vi "GetParam.vi"(8 "error in (no error)":errorcluster caption="entrée d'erreur (pas d'erreur)", 11 "GroupShuffleSplit.lvclass":refnum<class "GroupShuffleSplit.lvclass">) -> (0 "error out":errorcluster caption="sortie d'erreur", 2 "GroupShuffleSplit":T1={"n_splits"=5, "test_size"="0,2", "train_size"="None", "random_state"=-1} {"random_state" min=-1}, 3 "GroupShuffleSplit.lvclass":refnum<class "GroupShuffleSplit.lvclass">)   [LabVIEW 2020, in "GroupShuffleSplit.lvclass"]
doc: "Get Parameters"
uses:
  GroupShuffleSplit.lvclass
  GroupShuffleSplit.lvclass/GroupShuffleSplit.ctl
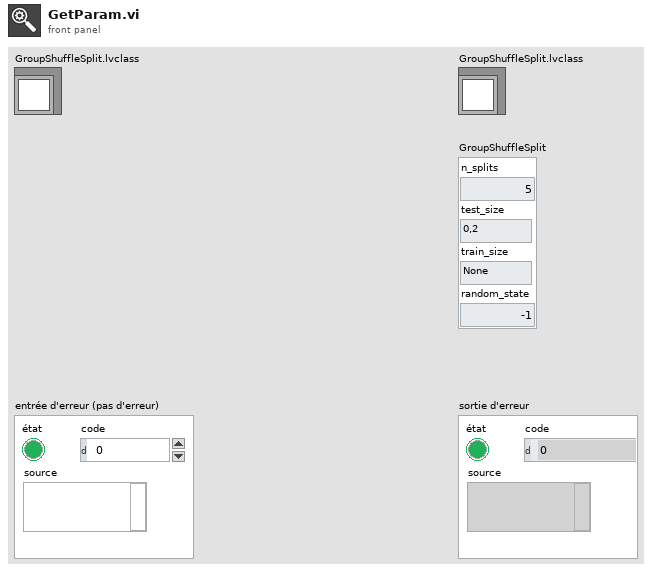
[diagram p1: front panel]
types:
  T1 = cluster{"n_splits":i32, "test_size":string, "train_size":string, "random_state":i32}
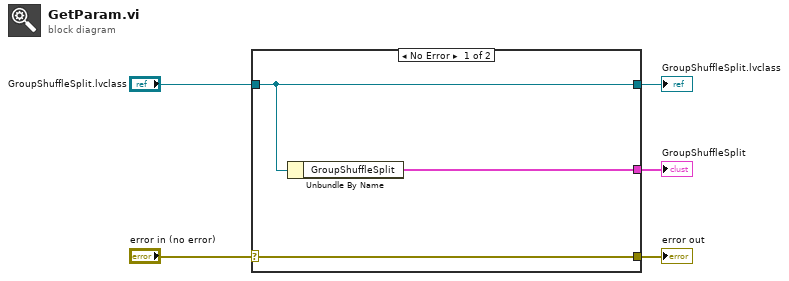
[diagram p0: block diagram]
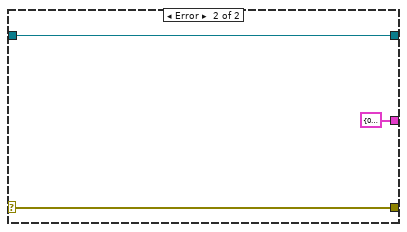
[diagram p2: hidden frame]
diagram:
  n1 = case shown="No Error" "error in (no error)" {
    selector: "error in (no error)" -> [w8 w10]
    tunnel: [w8 w10] -> w4
    tunnel: [w7 w11] -> w2
    tunnel: "GroupShuffleSplit.lvclass" -> [w7 w11]
    tunnel: [w6 T1 {"n_splits"=0, "test_size"="", "train_size"="", "random_state"=0} ("GroupShuffleSplit")] -> w1
    frame No Error {
      n2 = Unbundle By Name(w7) -> ("GroupShuffleSplit"=w6:T1)
    }
    frame Error {
    }
  }
  "error out" <- w4
  "GroupShuffleSplit.lvclass" <- w2
  "GroupShuffleSplit" <- w1
